vi "move relative.vi"(9 "error in (no error)":errorcluster, 10 "reference":refnum<k7>, 11 "relative displacment":sgl) -> (0 "reference out":refnum<k7>, 1 "error out":errorcluster, 2 "Current Position":sgl)   [LabVIEW 2011]
panel:
  out "MoveRelativeEx":i32
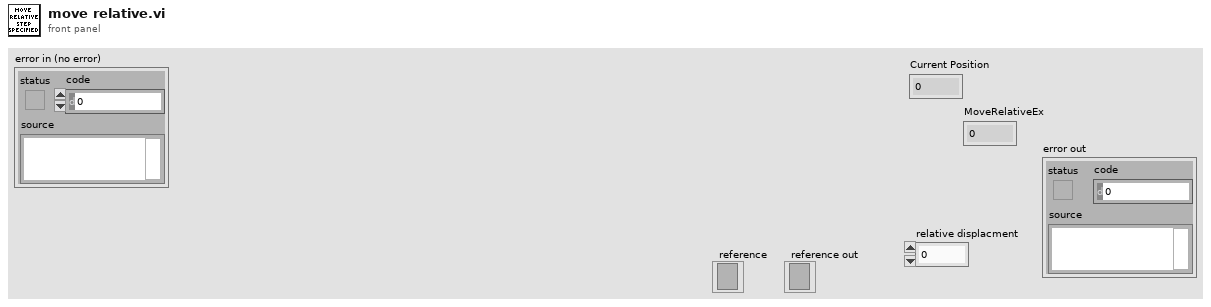
[diagram p1: front panel]
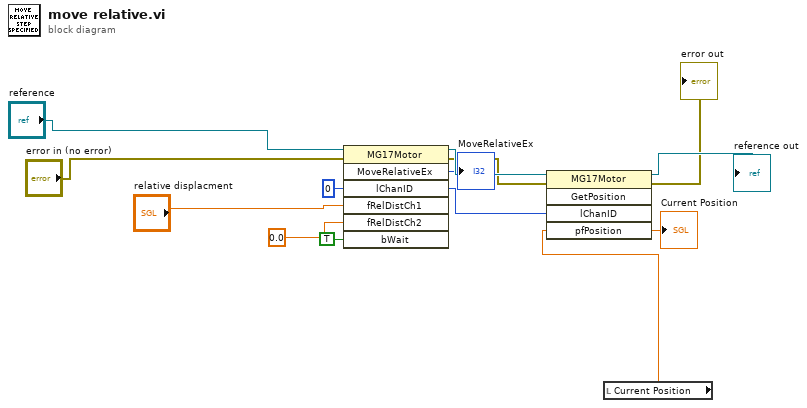
[diagram p0: block diagram]
diagram:
  n1 = invoke class="MG17Motor" method="MoveRelativeEx"(reference="reference", error in="error in (no error)", "lChanID"=0, "fRelDistCh1"="relative displacment", "fRelDistCh2"=sgl 0.0, "bWait"=TRUE) -> (reference out=w12:refnum<k7>, error out=w5:errorcluster, "MoveRelativeEx"=→"MoveRelativeEx":i32, "lChanID"=w10:i32)  [unwired: 1 in, 3 out]
  n2 = local read "Current Position"() -> (w3:sgl)
  n3 = invoke class="MG17Motor" method="GetPosition"(reference=w12, error in=w5, "lChanID"=w10, "pfPosition"=w3) -> (reference out=→"reference out":refnum<k7>, error out=→"error out":errorcluster, "pfPosition"=→"Current Position":sgl)  [unwired: 1 in, 2 out]
